vi "三维参数表面.vi"() -> ()   [LabVIEW 2010]
uses:
  <vilib>/Platform/NI_3dgraph.lvlib
panel:
  in  "三维参数曲面":refnum<k7>(container)
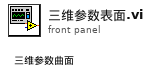
[diagram p1: front panel]
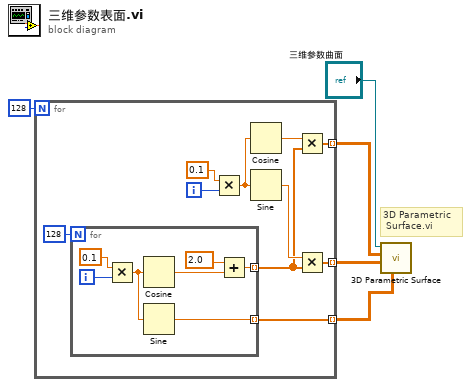
[diagram p0: block diagram]
diagram:
  # "3D Parametric\n Surface.vi"
  n1 = for {
    N: 128 -> [_]
    tunnel: [w6] -> w3 mode=indexing
    tunnel: [w10] -> w2 mode=indexing
    tunnel: [w13] -> w1 mode=indexing
    i -> [w11]
    n2 = for {
      N: 128 -> [_]
      tunnel: [w20] -> w7 mode=indexing
      tunnel: [w21] -> w13 mode=indexing
      i -> [w18]
      n3 = Multiply(x=0.1, y=w18) -> (x*y=w17:dbl)
      n4 = Cosine(x=w17) -> (cos(x)=w22:dbl)
      n5 = Sine(x=w17) -> (sin(x)=w21:dbl)
      n6 = Add(x=2.0, y=w22) -> (x+y=w20:dbl)
    }
    n7 = Multiply(x=0.1, y=w11) -> (x*y=w14:dbl)
    n8 = Cosine(x=w14) -> (cos(x)=w9:dbl)
    n9 = Sine(x=w14) -> (sin(x)=w8:dbl)
    n10 = Multiply(x=w9, y=w7) -> (x*y=w6:dbl[])
    n11 = Multiply(x=w8, y=w7) -> (x*y=w10:dbl[])
  }
  n12 = call <vilib>:"3D Parametric Surface.vi"("z matrix"=w1, "y matrix"=w2, "x matrix"=w3, "3D graph"="三维参数曲面") -> ()  [unwired: 6 in, 2 out]
